vi "3_STAGE.vi"(8 "Dataflow In":errorcluster) -> (0 "Dataflow Out":errorcluster)   [LabVIEW 2019]
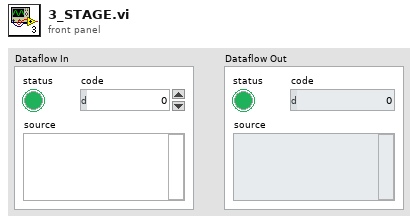
[diagram p1: front panel]
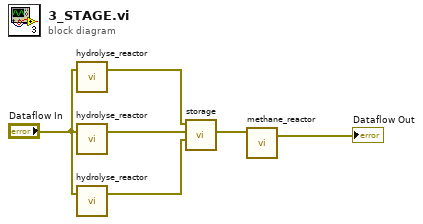
[diagram p0: block diagram]
diagram:
  n1 = call "hydrolyse_reactor.vi"("Dataflow In"="Dataflow In") -> ("Dataflow Out"=w3:errorcluster)  [unwired: 2 in]
  n2 = call "hydrolyse_reactor.vi"("Dataflow In"="Dataflow In") -> ("Dataflow Out"=w2:errorcluster)  [unwired: 2 in]
  n3 = call "hydrolyse_reactor.vi"("Dataflow In"="Dataflow In") -> ("Dataflow Out"=w1:errorcluster)  [unwired: 2 in]
  n4 = call "storage.vi"("Dataflow In #3"=w1, "Dataflow In #2"=w2, "Dataflow In #1"=w3) -> ("Dataflow Out"=w4:errorcluster)  [unwired: 8 in]
  n5 = call "methane_reactor.vi"("Dataflow In"=w4) -> ("Dataflow Out"=→"Dataflow Out":errorcluster)  [unwired: 4 in]
